vi "Analog Output.vi"(8 "error in (no error)":errorcluster, 11 "Analog Output in":refnum<class "Analog Output.lvclass">) -> (0 "error out":errorcluster, 3 "Analog Output out":refnum<class "Analog Output.lvclass">)   [LabVIEW 2017, in "Analog Output.lvclass"]
uses:
  Analog Output.lvclass
  <vilib>/DAQmx/create/channels.llb/DAQmx Create Channel (AO-Voltage-Basic).vi
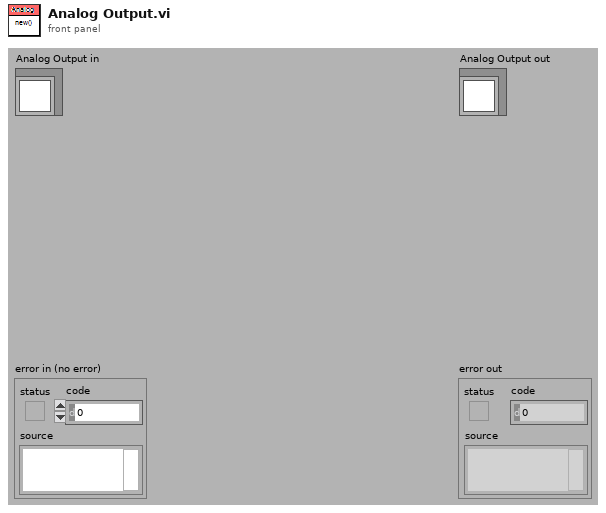
[diagram p1: front panel]
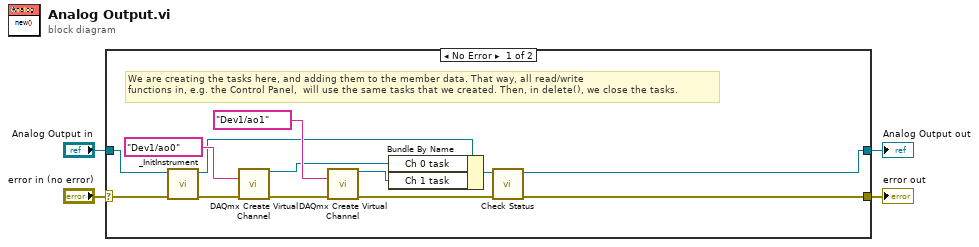
[diagram p0: block diagram]
diagram:
  n1 = case shown="No Error" "error in (no error)" {
    selector: "error in (no error)" -> [w16 w19]
    tunnel: [w14 w19] -> w3
    tunnel: [w15 w18] -> w1
    tunnel: "Analog Output in" -> [w17 w18]
    frame No Error {
      # "We are creating the tasks here, and adding them to the member data. That way, all read/write \nfunctions in, e.g. the Control Panel,  will use the same tasks that we created. Then, in delete(), we close the tasks."
      n2 = call-dynamic "_InitInstrument.vi"("error in (no error)"=w16, "Instrument in"=w17) -> ("error out"=w6:errorcluster, "Instrument out"=w11:refnum<class "Analog Output.lvclass">)  [unwired: 4 in, 4 out]
      n3 = call-poly <vilib>:"DAQmx Create Virtual Channel.vi"("physical channels"=tag "Dev1/ao0", "error in"=w6) -> ("task out"=w9:refnum<k21>, "error out"=w7:errorcluster)  [unwired: 12 in]
      n4 = call-poly <vilib>:"DAQmx Create Virtual Channel.vi"("physical channels"=tag "Dev1/ao1", "error in"=w7) -> ("task out"=w8:refnum<k21>, "error out"=w5:errorcluster)  [unwired: 12 in]
      n5 = Bundle By Name(cluster=w11, "Ch 0 task"=w9, "Ch 1 task"=w8) -> (w10:refnum<class "Analog Output.lvclass">)
      n6 = call-dynamic "Check Status.vi"("error in (no error)"=w5, "Analog Output in"=w10) -> ("error out"=w14:errorcluster, "Analog Output out"=w15:refnum<class "Analog Output.lvclass">)  [unwired: 6 in, 2 out]
    }
    frame Error {
    }
  }
  "error out" <- w3
  "Analog Output out" <- w1
